vi "Create Voice Sentence.vi"(7 "Description":string, 11 "Number":dbl) -> (3 "Voice Reporting Sentence":string)   [LabVIEW 2014]
doc: "This VI builds an english sentence out of a description and number.\n\nUsed with the voice reporting functionality of the ground station CO-PILOT."
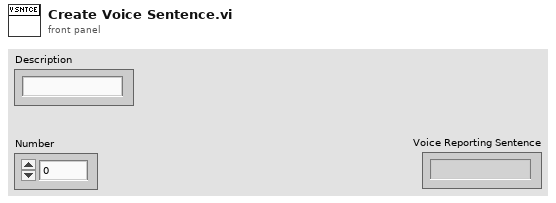
[diagram p1: front panel]
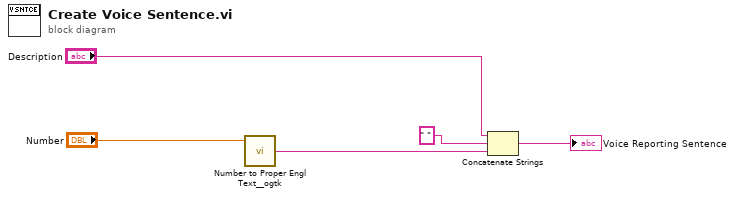
[diagram p0: block diagram]
diagram:
  n1 = call <userlib>:"Number to Proper Engl Text__ogtk.vi"("Numeric"="Number") -> ("String"=w5:string)  [unwired: 4 in]
  n2 = Concatenate Strings("Description", " " ("string"), w5) -> (→"Voice Reporting Sentence":string)
